vi "Script Init Values.vi"(4 "Special Terminals":T1={"Action"=-1, "Init"=-1, "Tag"=-1, "State in"=-1, "State out"=-1, "Error"=-1}, 8 "error in (no error)":errorcluster, 10 "Grouped Terminals":T3, 11 "Refs in":T2) -> (0 "error out":errorcluster, 3 "Refs":T2)   [LabVIEW 2020, in "FlexBlocks.lvlib"]
uses:
  FlexBlocks.lvlib
  Grouped Terminals.ctl
  Terminal Group.ctl
  Terminal Config.ctl
  Type Descriptor.ctl
  Terminal Direction.ctl
  Value Mode.ctl
  Special Terminal.ctl
  Terminal Mode.ctl
  Scripting Refs.ctl
  Special Terminal Indices.ctl
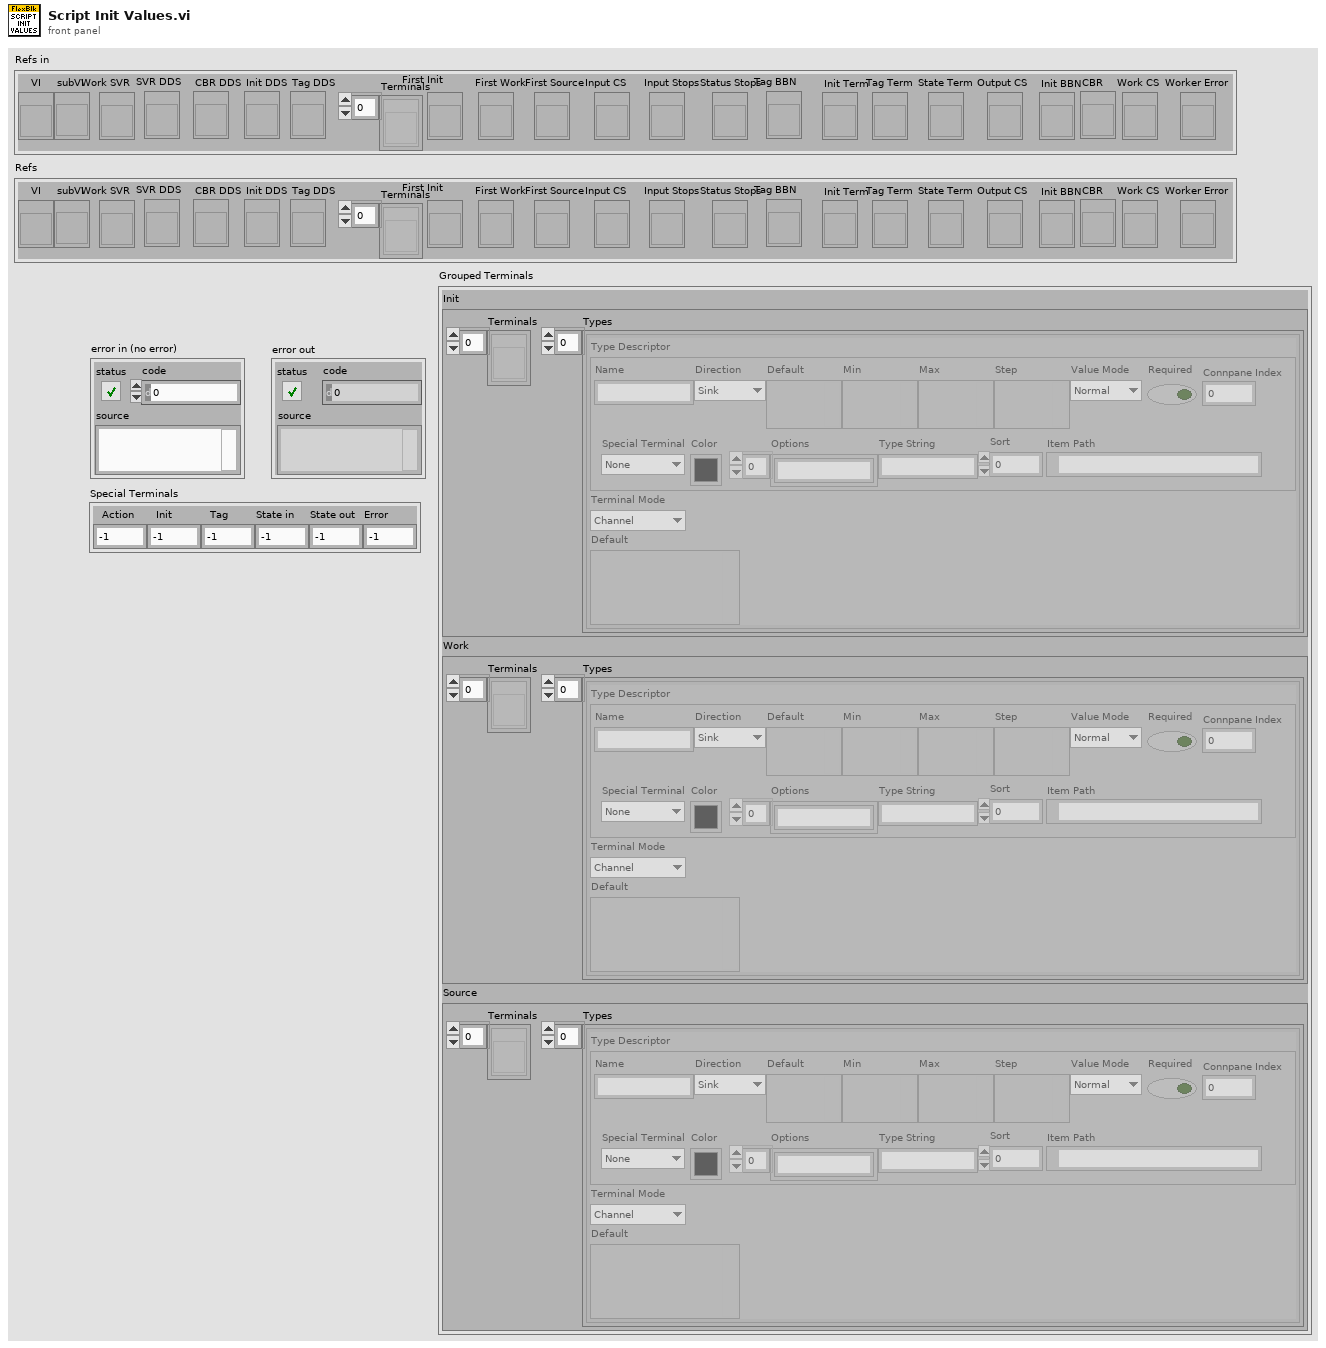
[diagram p1: front panel]
types:
  T1 = typedef "FlexBlocks.lvlib/Special Terminal Indices.ctl" = cluster{"Action":i32, "Init":i32, "Tag":i32, "State in":i32, "State out":i32, "Error":i32}
  T2 = typedef "FlexBlocks.lvlib/Scripting Refs.ctl" = cluster{"VI":refnum<vi>, "subVI":refnum<vi>, "Work SVR":refnum<vi>, "SVR DDS":refnum<vi>, "CBR DDS":refnum<vi>, "Init DDS":refnum<vi>, "Tag DDS":refnum<vi>, "Terminals":refnum<vi>[], "First Init":refnum<vi>, "First Work":refnum<vi>, "First Source":refnum<vi>, "Input CS":refnum<vi>, "Input Stops":refnum<vi>, "Status Stops":refnum<vi>, "Tag BBN":refnum<vi>, "Init Term":refnum<vi>, "Tag Term":refnum<vi>, "State Term":refnum<vi>, "Output CS":refnum<vi>, "Init BBN":refnum<vi>, "CBR":refnum<vi>, "Work CS":refnum<vi>, "Worker Error":refnum<vi>}
  T3 = typedef "FlexBlocks.lvlib/Grouped Terminals.ctl" = cluster{"Init":T4, "Work":T4, "Source":T4}
  T4 = typedef "FlexBlocks.lvlib/Terminal Group.ctl" = cluster{"Terminals":refnum<vi>[], "Types":T5[]}
  T5 = typedef "FlexBlocks.lvlib/Terminal Config.ctl" = cluster{"Type Descriptor":T6, "Terminal Mode":T10, "Default":variant}
  T6 = typedef "FlexBlocks.lvlib/Type Descriptor.ctl" = cluster{"Name":string, "Direction":T7, "Default":variant, "Min":variant, "Max":variant, "Step":variant, "Value Mode":T8, "Required":bool, "Connpane Index":i32, "Special Terminal":T9, "Color":u32, "Options":string[], "Type String":string, "Sort":i32, "Item Path":path}
  T7 = typedef "FlexBlocks.lvlib/Terminal Direction.ctl" = enum16{"Sink", "Source"}
  T8 = typedef "FlexBlocks.lvlib/Value Mode.ctl" = enum16{"Normal", "Range", "Select"}
  T9 = typedef "FlexBlocks.lvlib/Special Terminal.ctl" = enum16{"None", "Action", "Init", "Tag", "State in", "State out", "Error"}
  T10 = typedef "FlexBlocks.lvlib/Terminal Mode.ctl" = enum16{"Channel", "Config", "Value", "Control Ref"}
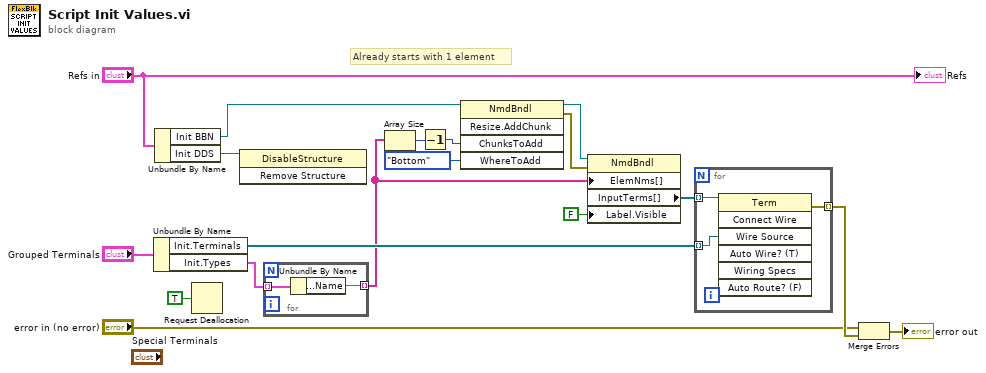
[diagram p0: block diagram]
diagram:
  # "Already starts with 1 element"
  n1 = Unbundle By Name("Grouped Terminals") -> ("Init.Terminals"=w14:refnum<vi>[], "Init.Types"=w7:T5[])
  n2 = Unbundle By Name("Refs in") -> ("Init BBN"=w8:refnum<vi>, "Init DDS"=w15:refnum<vi>)
  n3 = Request Deallocation(TRUE ("flag")) -> ()
  n4 = invoke class="DisableStructure" method="Remove Structure"(reference=w15) -> ()  [unwired: 2 in, 3 out]
  n5 = for {
    tunnel: w7 -> [w20] mode=indexing
    tunnel: [w19] -> w6 mode=indexing
    n6 = Unbundle By Name(w20) -> ("Type Descriptor.Name"=w19:string)
  }
  n7 = Array Size(array=w6) -> (size(s)=w12:i32)
  n8 = Decrement(x=w12) -> (x-1=w11:i32)
  n9 = invoke class="NmdBndl" method="Resize.AddChunk"(reference=w8, "ChunksToAdd"=w11, "WhereToAdd"=enum8{"Bottom", "Top"}."Bottom" ("Where To Add")) -> (reference out=w4:refnum<vi>, error out=w10:errorcluster)  [unwired: 2 in, 3 out]
  n10 = property class="NmdBndl"(reference=w4, error in=w10, "ElemNms[]"=w6, "Label.Visible"=FALSE) -> ("InputTerms[]"=w5:refnum<vi>[])  [unwired: 2 out]
  n11 = for {
    tunnel: w14 -> [w22] mode=indexing
    tunnel: w5 -> [w23] mode=indexing
    tunnel: [w21] -> w3 mode=indexing
    n12 = invoke class="Term" method="Connect Wire"(reference=w23, "Wire Source"=w22) -> (error out=w21:errorcluster)  [unwired: 5 in, 6 out]
  }
  n13 = Merge Errors("error in (no error)", w3) -> (→"error out":errorcluster)
  "Refs" <- "Refs in"
